vi "数组极值.vi"() -> ()   [LabVIEW 2010]
panel:
  out "最小值位置":i32[](array[numeric])
  out "最小值":dbl format="%.2f"
  out "最大值位置":i32[](array[numeric])
  out "最大值":dbl format="%.2f"
  out "最小值位置":i32
  out "最小值":dbl format="%.2f"
  out "最大值位置":i32
  out "最大值":dbl format="%.2f"
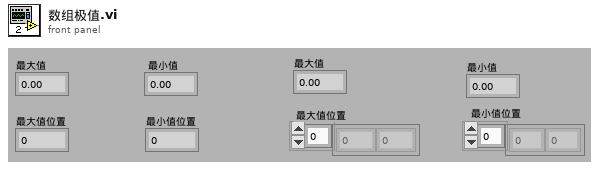
[diagram p1: front panel]
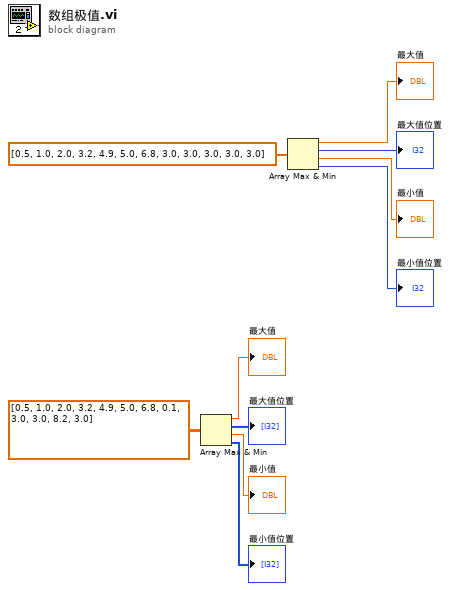
[diagram p0: block diagram]
diagram:
  n1 = Array Max & Min(array=dbl[][] [[0.5, 1.0, 2.0, 3.2], [4.9, 5.0, 6.8, 0.1], [3.0, 3.0, 8.2, 3.0]] ("output array")) -> (max value=→"最大值":dbl, max index (indices)=→"最大值位置":i32[], min value=→"最小值":dbl, min index (indices)=→"最小值位置":i32[])
  n2 = Array Max & Min(array=dbl[] [0.5, 1.0, 2.0, 3.2, 4.9, 5.0, 6.8, 3.0, 3.0, 3.0, 3.0, 3.0] ("Array")) -> (max value=→"最大值":dbl, max index (indices)=→"最大值位置":i32, min value=→"最小值":dbl, min index (indices)=→"最小值位置":i32)
